vi "KE622x -- Get Standard Event Enable Reg State.vi"(0 "VISA Resource In":refnum<visa-resource-name>, 1 "Error Query (T)?":bool=TRUE, 11 "error in (no error)":errorcluster) -> (4 "VISA Resource Out (dupl)":refnum<visa-resource-name>, 8 "KE622x Standard Event Enable Reg":T1, 15 "error out":errorcluster)   [LabVIEW 2009, in "Keithley 622x.lvlib"]
doc: "Returns the bits in the 'Standard Event Enable' register of the Status Model. Note that only the used (named) bits are returned."
uses:
  <instrlib>/Keithley 622x LV 2009/Keithley 622x.lvlib
  <instrlib>/Keithley 622x LV 2009/Utility/Status Registers/Typedefs/KE622x -- Standard Event Enable Reg State.ctl
panel:
  out "Reg Num (dec)":u16 format="%0d"
  out "Reg Num (binary)":u16 format="%016b"
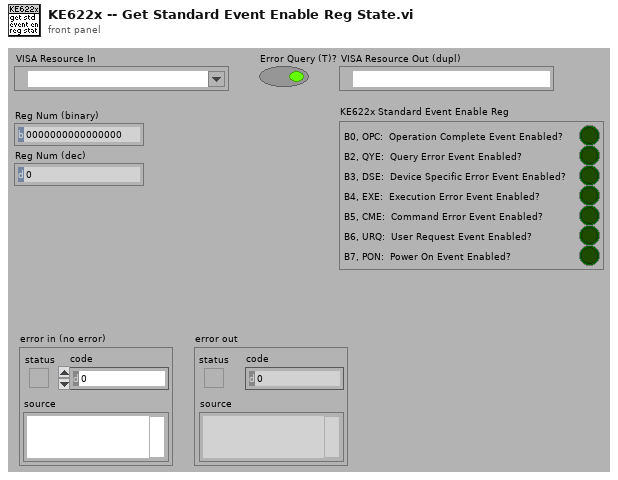
[diagram p1: front panel]
types:
  T1 = typedef "Keithley 622x.lvlib/KE622x -- Standard Event Enable Reg State.ctl" = cluster{"B0, OPC:  Operation Complete Event Enabled?":bool, "B2, QYE:  Query Error Event Enabled?":bool, "B3, DSE:  Device Specific Error Event Enabled?":bool, "B4, EXE:  Execution Error Event Enabled?":bool, "B5, CME:  Command Error Event Enabled?":bool, "B6, URQ:  User Request Event Enabled?":bool, "B7, PON:  Power On Event Enabled?":bool}
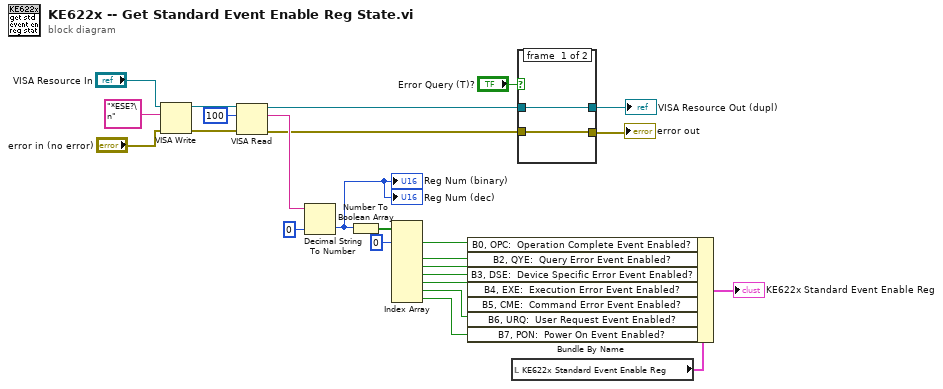
[diagram p0: block diagram]
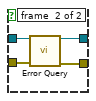
[diagram p2: hidden frame]
diagram:
  n1 = VISA Write(VISA resource name="VISA Resource In", write buffer="*ESE?\n", error in (no error)="error in (no error)") -> (VISA resource name out=w22:refnum<visa-resource-name>, error out=w21:errorcluster)  [unwired: 1 out]
  n2 = VISA Read(VISA resource name=w22, byte count=u32 100, error in (no error)=w21) -> (VISA resource name out=w3:refnum<visa-resource-name>, read buffer=w19:string, error out=w4:errorcluster)  [unwired: 1 out]
  n3 = Decimal String To Number(string=w19, default (0L)=u16 0 ("default (0 I32)")) -> (number=w13:u16)  [unwired: 2 out]
  "Reg Num (binary)" <- w13
  "Reg Num (dec)" <- w13
  n4 = Number To Boolean Array(number=w13) -> (Boolean array=w17:bool[])
  n5 = Index Array(array=w17, index #1=0 ("index")) -> (element #1=w14:bool, element #3=w12:bool, element #4=w11:bool, element #5=w10:bool, element #6=w9:bool, element #7=w8:bool, element #8=w7:bool)  [unwired: 7 in, 1 out]
  n6 = local read "KE622x Standard Event Enable Reg"() -> (w15:T1)
  n7 = Bundle By Name(cluster=w15, "B0, OPC:  Operation Complete Event Enabled?"=w14, "B2, QYE:  Query Error Event Enabled?"=w12, "B3, DSE:  Device Specific Error Event Enabled?"=w11, "B4, EXE:  Execution Error Event Enabled?"=w10, "B5, CME:  Command Error Event Enabled?"=w9, "B6, URQ:  User Request Event Enabled?"=w8, "B7, PON:  Power On Event Enabled?"=w7) -> (→"KE622x Standard Event Enable Reg":T1)
  n8 = case shown="True" "Error Query (T)?" {
    tunnel: w4 -> [w26 w31]
    tunnel: w3 -> [w27 w30]
    tunnel: [w26 w29] -> w1
    tunnel: [w27 w28] -> w2
    frame #0 {
    }
    frame #1 {
      n9 = call <instrlib>:"Error Query.vi"("VISA Resource In"=w30, "error in (no error)"=w31) -> ("VISA Resource Out (dupl)"=w28:refnum<visa-resource-name>, "error out"=w29:errorcluster)  [unwired: 10 in, 2 out]
    }
  }
  "VISA Resource Out (dupl)" <- w2
  "error out" <- w1
